vi "TCPIP Protocol FG.vi"(7 "Action":T1, 8 "error in (no error)":errorcluster, 10 "TCP/IP Config":T2={"IP Address"="localhost", "Port"=8888}, 11 "Device Item Ref in":T3 format="%.0x") -> (0 "error out":errorcluster, 2 "TCP/IP Config":T2={"IP Address"="localhost", "Port"=8888}, 3 "Item Ref out":T3 format="%.0x")   [LabVIEW 2015, in "Instrument Addon Shared.lvlib"]
uses:
  Instrument Addon Shared.lvlib
  <vilib>/NI Veristand/Custom Device API/Custom Device Item Ref.ctl
  Types/TCPIP Settings.ctl
  Types/FG Control.ctl
  <vilib>/NI Veristand/Custom Device API/Set Item Property (U32).vi
  <vilib>/NI Veristand/Custom Device API/Set Item Property (String).vi
  <vilib>/NI Veristand/Custom Device API/Get Item Property (U32).vi
  <vilib>/NI Veristand/Custom Device API/Get Item Property (String).vi
  Constants.vi
  <vilib>/NI VeriStand/Custom Device API/Custom Device API.lvlib
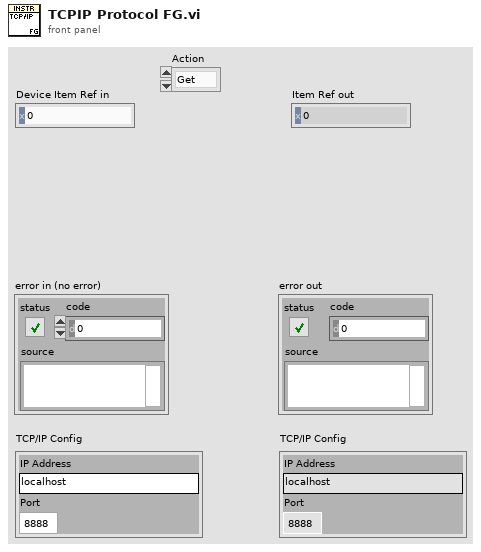
[diagram p1: front panel]
types:
  T1 = typedef "Instrument Addon Shared.lvlib/FG Control.ctl" = enum16{"Get", "Set"}
  T2 = typedef "Instrument Addon Shared.lvlib/TCPIP Settings.ctl" = cluster{"IP Address":string, "Port":u16}
  T3 = typedef "Custom Device API.lvlib/Custom Device Item Ref.ctl" = u64
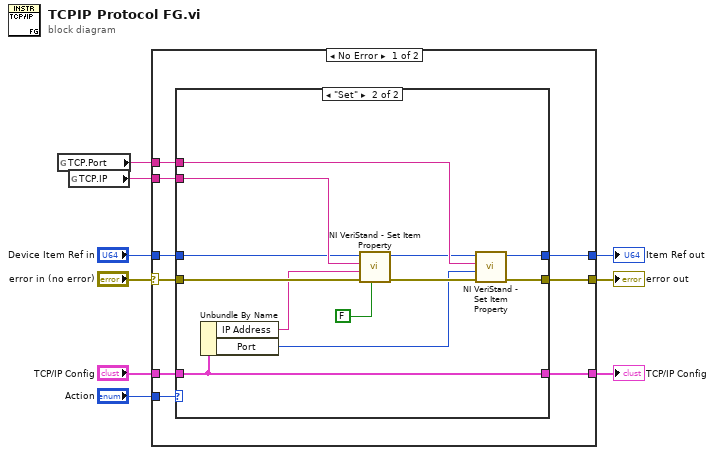
[diagram p0: block diagram]
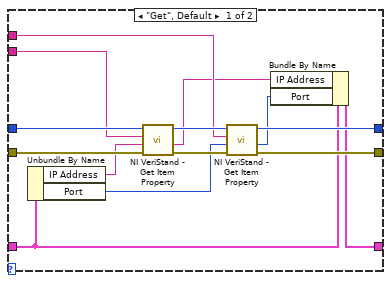
[diagram p2: hidden frame]
diagram:
  n1 = global read "Constants.vi" "TCP.Port"() -> (w1:string)
  n2 = global read "Constants.vi" "TCP.IP"() -> (w9:string)
  n3 = case shown="No Error" "error in (no error)" {
    selector: "error in (no error)" -> [w13 w47]
    tunnel: w9 -> [w18 _]
    tunnel: [w17 w45] -> w8
    tunnel: "Device Item Ref in" -> [w16 w45]
    tunnel: "TCP/IP Config" -> [w15 w46]
    tunnel: [w14 w47] -> w5
    tunnel: [w12 w46] -> w3
    tunnel: "Action" -> [w11 _]
    tunnel: w1 -> [w10 _]
    frame No Error {
      n4 = case shown="\"Set\"" w11 {
        tunnel: w18 -> [w30 w44]
        tunnel: [w25 w38] -> w17
        tunnel: w16 -> [w31 w43]
        tunnel: w15 -> [w22 w35]
        tunnel: [w27 w37] -> w14
        tunnel: w13 -> [w32 w42]
        tunnel: [w19 w35] -> w12
        tunnel: w10 -> [w26 w40]
        frame "Get", Default {
          n5 = Unbundle By Name(w22) -> ("IP Address"=w24:string, "Port"=w23:u16)
          n6 = call-poly <vilib>:"NI VeriStand - Get Item Property.vi"("error in (no error)"=w32, "Default Value"=w24, "Property Name"=w30, "Item Ref in"=w31) -> ("error out"=w28:errorcluster, "Value"=w21:string, "Item Ref out"=w29:T3)  [unwired: 4 in, 1 out]
          n7 = call-poly <vilib>:"NI VeriStand - Get Item Property.vi"("error in (no error)"=w28, "Default Value"=w23, "Property Name"=w26, "Item Ref in"=w29) -> ("error out"=w27:errorcluster, "Value"=w20:u32, "Item Ref out"=w25:T3)  [unwired: 4 in, 1 out]
          n8 = Bundle By Name(cluster=w22, "IP Address"=w21, "Port"=w20) -> (w19:T2)
        }
        frame "Set" {
          n9 = Unbundle By Name(w35) -> ("IP Address"=w34:string, "Port"=w33:u16)
          n10 = call-poly <vilib>:"NI VeriStand - Set Item Property.vi"("Binary String (T)"=FALSE, "error in (no error)"=w42, "Value"=w34, "Property Name"=w44, "Item Ref in"=w43) -> ("error out"=w36:errorcluster, "Item Ref out"=w39:T3)  [unwired: 4 in, 1 out]
          n11 = call-poly <vilib>:"NI VeriStand - Set Item Property.vi"("error in (no error)"=w36, "Value"=w33, "Property Name"=w40, "Item Ref in"=w39) -> ("error out"=w37:errorcluster, "Item Ref out"=w38:T3)  [unwired: 5 in, 1 out]
        }
      }
    }
    frame Error {
    }
  }
  "Item Ref out" <- w8
  "error out" <- w5
  "TCP/IP Config" <- w3
